vi "adam-DO-send-command.vi"(6 "Stop All":bool, 8 "error in (no error)":errorcluster, 9 "Channel Active":bool, 10 "Channel Number":dbl=1.0, 11 "VISA Refnum in":refnum<visa-resource-name>) -> (0 "error out":errorcluster, 1 "Desired State":bool, 3 "VISA Refnum out":refnum<visa-resource-name>, 4 "STOPPED":bool, 5 "Bytes Written":u32, 7 "command":string)   [LabVIEW 2021]
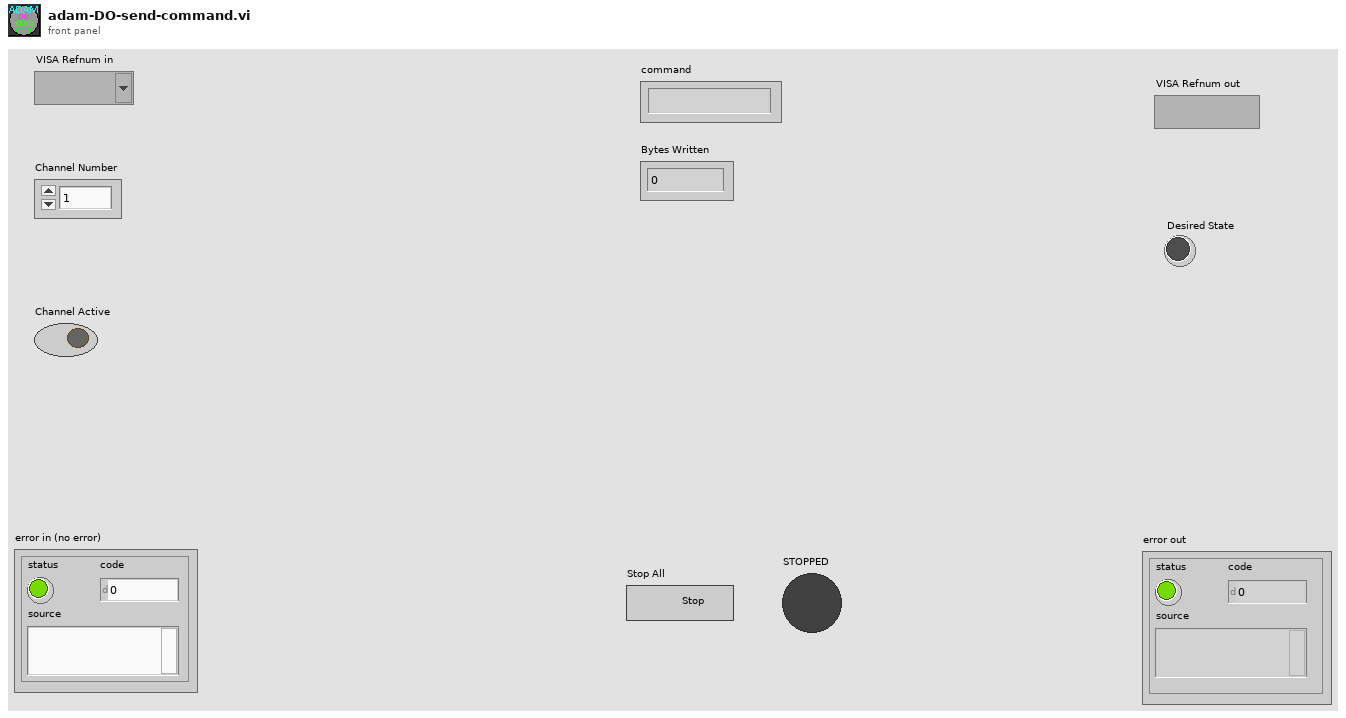
[diagram p1: front panel]
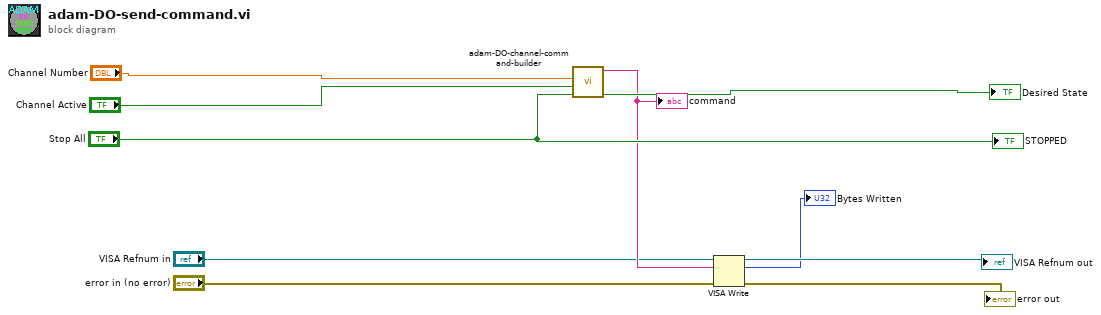
[diagram p0: block diagram]
diagram:
  n1 = call "adam-DO-channel-command-builder.vi"("Stop All"="Stop All", "Channel Active"="Channel Active", "Channel Number"="Channel Number") -> ("Desired State"=→"Desired State":bool, "concatenated command"=w8:string)  [unwired: 7 in]
  "command" <- w8
  n2 = VISA Write(VISA resource name="VISA Refnum in", write buffer=w8, error in (no error)="error in (no error)") -> (VISA resource name out=→"VISA Refnum out":refnum<visa-resource-name>, return count=→"Bytes Written":u32, error out=→"error out":errorcluster)
  "STOPPED" <- "Stop All"
